vi "m_getunits.vi"(2 "error in (no error)":errorcluster) -> (0 "error out":errorcluster, 1 "Wavelength Units":u16(ring) items=["nanometer", "micrometer", "wavenumber"])   [LabVIEW 2017]
doc: "Queries the wavelength units in use from the monochromator"
panel:
  out "Units":u16(ring) items=["NM", "UM", "WN"]
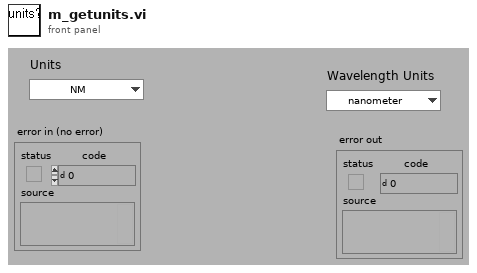
[diagram p1: front panel]
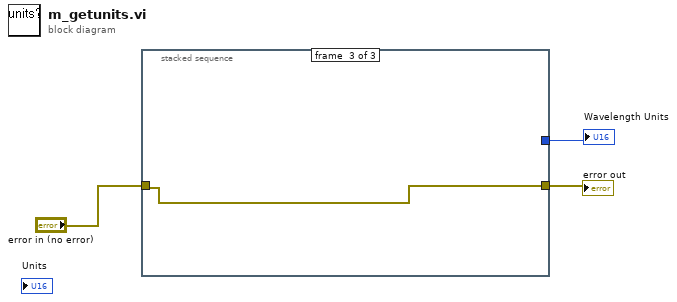
[diagram p0: block diagram]
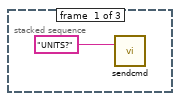
[diagram p2: hidden frame]
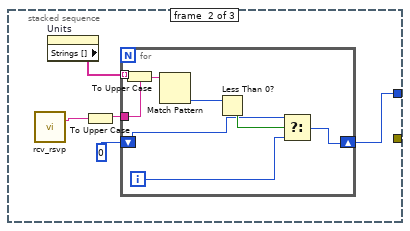
[diagram p3: hidden frame]
diagram:
  n1 = stacked-sequence {
    tunnel: "error in (no error)" -> [_ _ w18]
    tunnel: [_ _ w18] -> w2
    tunnel: [_ w7 _] -> w1
    frame #0 {
      n2 = call "sendcmd.vi"("command in"="UNITS?") -> ()  [unwired: 2 in, 1 out]
    }
    frame #1 {
      n3 = call "rcv_rsvp.vi"() -> ("response string"=w5:string)  [unwired: 2 in, 1 out]
      n4 = property on="Units" class="Ring (strict)"() -> ("Strings []"=w9:string[])  [unwired: 2 in, 2 out]
      n5 = To Upper Case(1:w5) -> (0:w6:string)
      n6 = for {
        tunnel: w9 -> [w15] mode=indexing
        tunnel: w6 -> [w17]
        shift-right: [w11] -> w7
        shift-left: 0 -> [w13]
        i -> [w12]
        n7 = To Upper Case(1:w15) -> (0:w10:string)
        n8 = Match Pattern(string=w17, regular expression=w10) -> (offset past match=w16:i32)  [unwired: 1 in, 3 out]
        n9 = Less Than 0?(x=w16) -> (x < 0?=w14:bool)
        n10 = Select(t=w13, s=w14, f=w12) -> (s? t:f=w11:i32)
      }
    }
    frame #2 {
    }
  }
  "error out" <- w2
  "Wavelength Units" <- w1
